vi "VI-Fix Labels.vi"(0 "VI in":refnum<vi>, 11 "error in (no error)":errorcluster) -> (4 "VI out":refnum<vi>, 15 "error out":errorcluster)   [LabVIEW 2015]
uses:
  <vilib>/Utility/traverseref.llb/TRef TravTarget.ctl
  <vilib>/Utility/traverseref.llb/VI Scripting - Traverse.lvlib
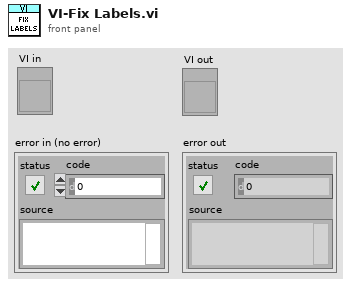
[diagram p1: front panel]
types:
  T1 = typedef "TRef TravTarget.ctl" = enum16{"FP", "BD", "Other"}
  T2 = typedef "LVRectTypeDef.ctl" = cluster{"Left":i16, "Top":i16, "Right":i16, "Bottom":i16}
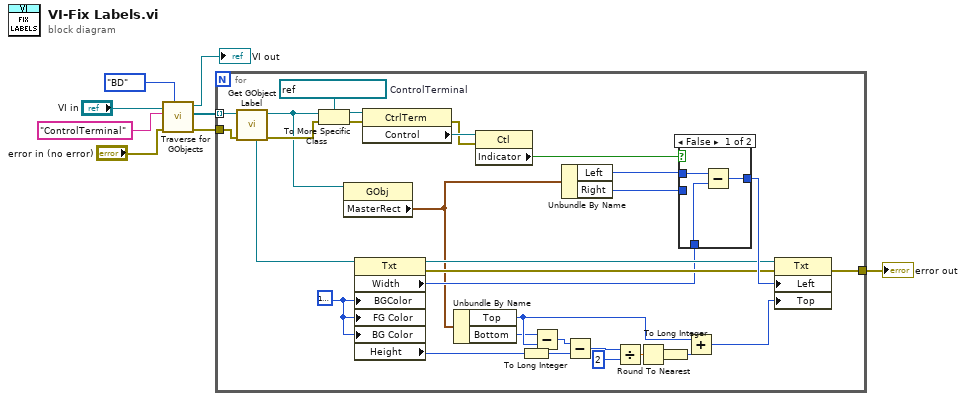
[diagram p0: block diagram]
diagram:
  n1 = call <vilib>:"Traverse for GObjects.vi"("Traverse Target"=TRef_TravTarget."BD", "error in (no error)"="error in (no error)", "Class Name"="ControlTerminal", "VI Refnum"="VI in") -> ("error out"=w2:errorcluster, "References"=w7:refnum<vi>[], "dup VI Refnum"=→"VI out":refnum<vi>)  [unwired: 4 in, 1 out]
  n2 = for {
    tunnel: w7 -> [w20] mode=indexing
    tunnel: w2 -> [w35]
    tunnel: [w26] -> w1
    w38 = refnum<vi> refnum  # ControlTerminal
    w22 = u32 16777216
    n3 = call <vilib>:"Get GObject Label.vi"("error in (no error)"=w35, "GObject"=w20) -> ("error out"=w34:errorcluster, "dup GObject"=w16:refnum<vi>, "Label Reference"=w39:refnum<vi>)  [unwired: 5 in, 2 out]
    n4 = To More Specific Class(target class=w38, reference=w16, error in=w34) -> (specific class reference=w37:refnum<vi>, error out=w33:errorcluster)
    n5 = property class="GObj"(reference=w16) -> ("MasterRect"=w17:T2)  [unwired: 1 in, 2 out]
    n6 = property class="Txt"(reference=w39, "BGColor"=w22, "FG Color"=w22, "BG Color"=w22) -> (reference out=w24:refnum<vi>, error out=w23:errorcluster, "Width"=w21:u32, "Height"=w31:u32)  [unwired: 1 in]
    n7 = property class="CtrlTerm"(reference=w37, error in=w33) -> (error out=w32:errorcluster, "Control"=w36:refnum<vi>)  [unwired: 1 out]
    n8 = Unbundle By Name(w17) -> ("Top"=w14:i16, "Bottom"=w13:i16)
    n9 = property class="Ctl"(reference=w36, error in=w32) -> ("Indicator"=w27:bool)  [unwired: 2 out]
    n10 = To Long Integer(number=w31) -> (32bit integer=w11:i32)
    n11 = Subtract(x=w13, y=w14) -> (x-y=w15:i16)
    n12 = Unbundle By Name(w17) -> ("Left"=w18:i16, "Right"=w19:i16)
    n13 = Subtract(x=w15, y=w11) -> (x-y=w30:i32)
    n14 = Divide(x=w30, y=2) -> (x/y=w28:dbl)
    n15 = Round To Nearest(number=w28) -> (nearest integer value=w10:dbl)
    n16 = To Long Integer(number=w10) -> (32bit integer=w9:i32)
    n17 = case shown="False" w27 {
      tunnel: w18 -> [w41 _]
      tunnel: w19 -> [_ w43]
      tunnel: [w42 w43] -> w25
      tunnel: w21 -> [w40 _]
      frame False {
        n18 = Subtract(x=w41, y=w40) -> (x-y=w42:u32)
      }
      frame True {
      }
    }
    n19 = Add(x=w14, y=w9) -> (x+y=w12:i32)
    n20 = property class="Txt"(reference=w24, error in=w23, "Left"=w25, "Top"=w12) -> (error out=w26:errorcluster)  [unwired: 1 out]
  }
  "error out" <- w1
